vi "Leap Key Tap Gesture.vi"() -> ()   [LabVIEW 2014, in "LMH-Leap.lvlib"]
doc: "This example demonstrates how to read the position of a key tap gesture using the Leap Motion Controller."
uses:
  vi.lib/MakerHub/Leap/LMH-Leap.lvlib
  vi.lib/MakerHub/Leap/Public/Gestures/Key Tap/Instance VIs/Read 1 Key Tap Position.vi
panel:
  out "X Z Key Tap Position":cluster{"X":sgl, "Z":sgl}[](graph)
  out "Last Key Tap Position":cluster{"X":sgl, "Y":sgl, "Z":sgl}
  in  "Stop Button":bool
  # "Leap Key Tap Gesture Example\n\nThis example demonstrates how to read the position of a key tap gesture using the Leap Motion Controller.\n\nInstructions\n1. Connect the Leap Motion Controller to the host computer.\n2. Click the Run Arrow.\n3. Make a key tap gesture above the Leap and notice the position indicated on the graph below."
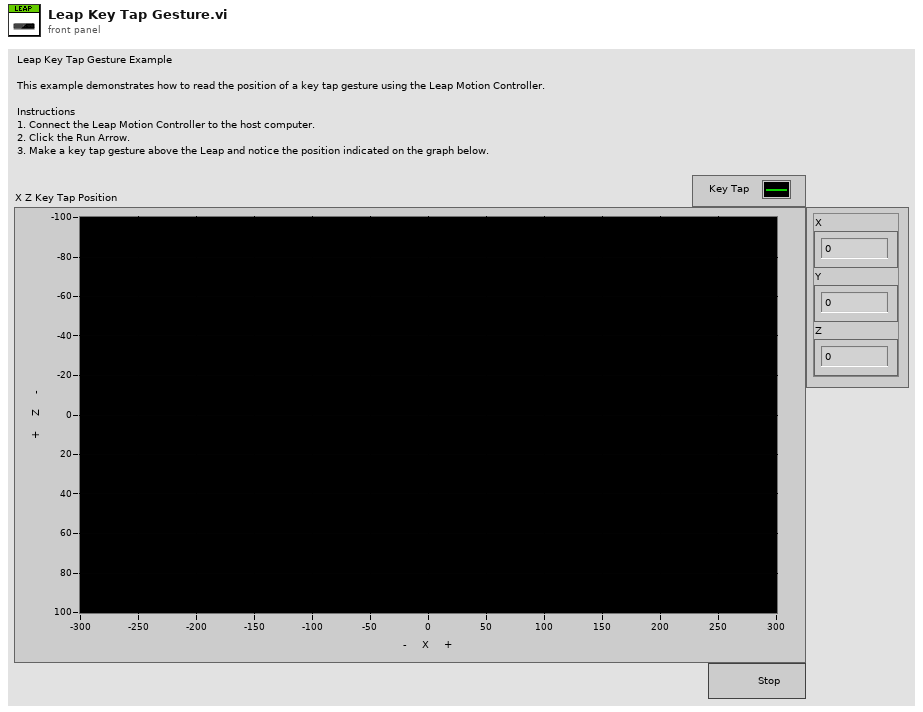
[diagram p1: front panel]
types:
  T1 = typedef "LMH-Leap.lvlib/Leap Handle.ctl" = cluster{"LeapCSharp":refnum<k24>}
  T2 = typedef "LMH-Leap.lvlib/Gesture State.ctl" = enum16{"Invalid", "Start", "Update", "Stop"}
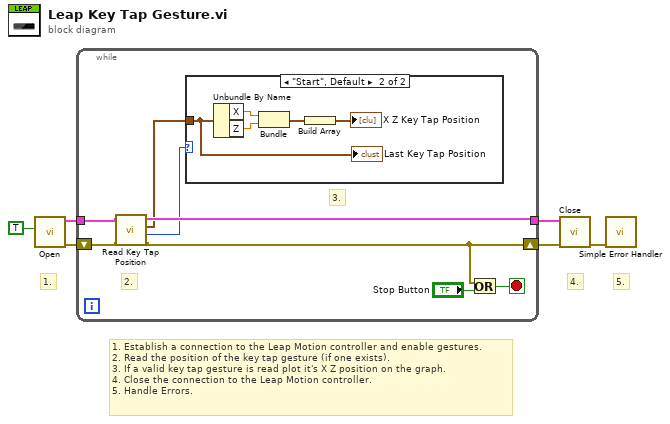
[diagram p0: block diagram]
diagram:
  # "5."
  # "4."
  # "1."
  # "1. Establish a connection to the Leap Motion controller and enable gestures.\n2. Read the position of the key tap gesture (if one exists).\n3. If a valid key tap gesture is read plot it's X Z position on the graph.\n4. Close the connection to the Leap Motion controller.\n5. Handle Errors."
  n1 = call "Open.vi"("Enable Gestures? (T)"=TRUE) -> ("Error Out"=w4:errorcluster, "Leap Handle"=w6:T1)  [unwired: 9 in]
  n2 = while {
    tunnel: w6 -> [w12]
    shift-right: [w11] -> w5
    shift-left: w4 -> [w10]
    tunnel: [w9] -> w2
    stop <- w14 stop-if-true
    # "3."
    # "2."
    n3 = call-poly "Read Key Tap Position.vi"("Error In"=w10, "Leap Handle"=w12) -> ("Error Out"=w11:errorcluster, "Key Tap Status"=w8:T2, "Key Tap Position"=w7:cluster{"X":sgl, "Y":sgl, "Z":sgl}, "Leap Handle"=w9:T1)  [unwired: 6 in]
    n4 = case shown="\"Start\", Default" w8 {
      tunnel: w7 -> [_ w19]
      frame "Invalid" {
      }
      frame "Start", Default {
        n5 = Unbundle By Name(w19) -> ("X"=w18:sgl, "Z"=w17:sgl)
        n6 = Bundle("X"=w18, "Z"=w17) -> (w16:cluster{"X":sgl, "Z":sgl})  [unwired: 1 in]
        n7 = Build Array(w16) -> (→"X Z Key Tap Position":cluster{"X":sgl, "Z":sgl}[])
        "Last Key Tap Position" <- w19
      }
    }
    n8 = Or(x=w11, y="Stop Button") -> (x .or. y?=w14:bool)
  }
  n9 = call "Close.vi"("Error In"=w5, "Leap Handle"=w2) -> ("Error Out"=w1:errorcluster)  [unwired: 9 in]
  n10 = call <vilib>:"Simple Error Handler.vi"("error in (no error)"=w1) -> ()  [unwired: 4 in, 5 out]
